vi "Pr650_K2400_Measure09.vi"(5 "error in":errorcluster, 6 "Volt":string, 7 "Device Name":string="OLED", 8 "Path":path=path "C:/temp", 9 "Keithly2400 Address":string, 10 "Port":i32(ring) items=["COM1", "COM2"]) -> (0 "error out(measure and off)":errorcluster, 1 "1931 CIE x":string, 2 "L: Cd/m^2":string, 3 "Keithley Data":string, 4 "1931 CIE y":string)   [LabVIEW 2009]
panel:
  in  "分支常量\n（见即时帮助）":bool
  out "string read":string
  out "error out(setup and on)":errorcluster
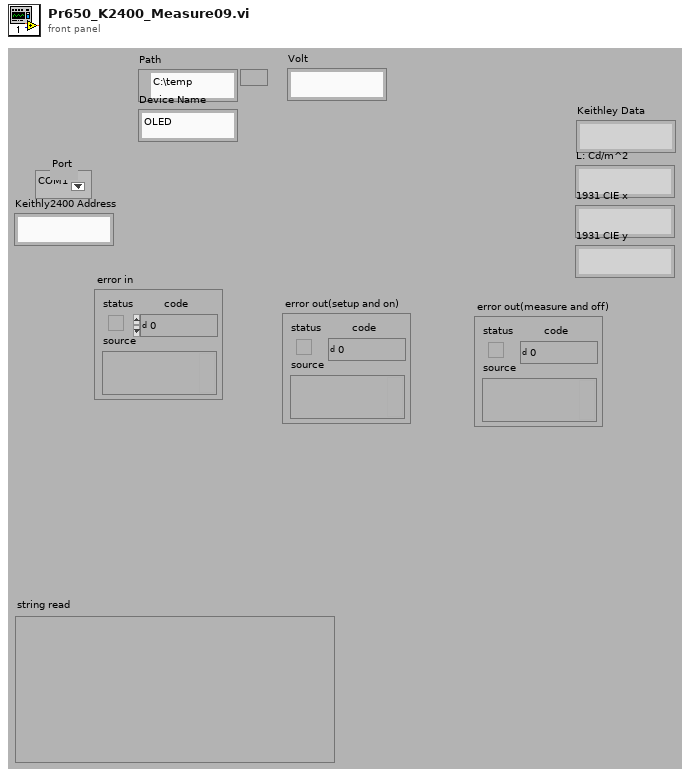
[diagram p1: front panel]
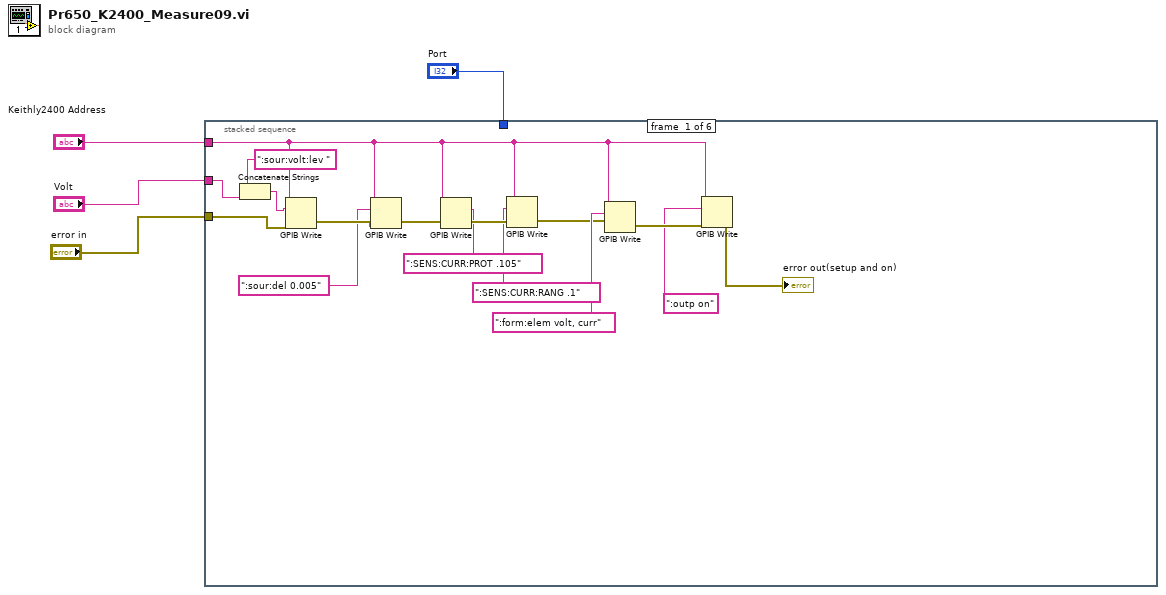
[diagram p0: block diagram]
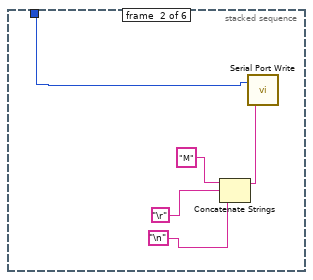
[diagram p2: hidden frame]
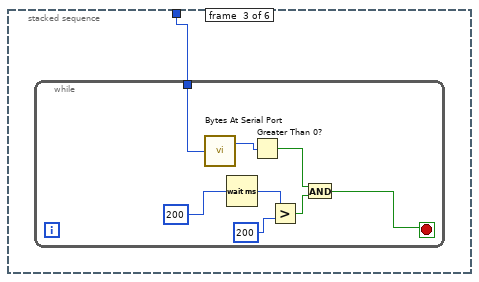
[diagram p3: hidden frame]
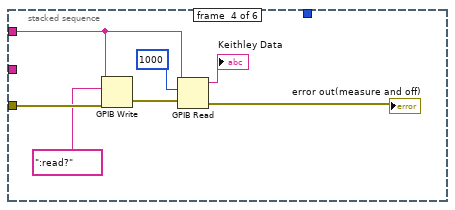
[diagram p4: hidden frame]
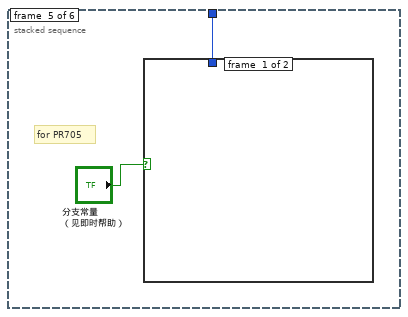
[diagram p5: hidden frame]
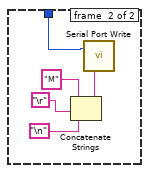
[diagram p6: hidden frame]
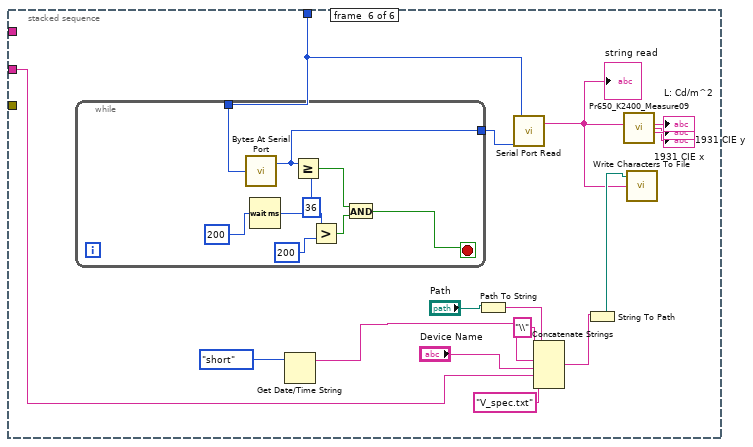
[diagram p7: hidden frame]
diagram:
  n1 = stacked-sequence {
    tunnel: "Port" -> [_ w22 w26 _ w43 w51]
    tunnel: "error in" -> [w20 _ _ w41 _ _]
    tunnel: "Keithly2400 Address" -> [w10 _ _ w36 _ _]
    tunnel: "Volt" -> [w14 _ _ _ _ w54]
    frame #0 {
      n2 = Concatenate Strings(":sour:volt:lev ", w14) -> (w12:string)
      n3 = GPIB Write(0:w10, 1:w12, 3:w20) -> (6:w19:errorcluster)  [unwired: 2 in, 1 out]
      n4 = GPIB Write(0:w10, 1:":sour:del 0.005" ("data"), 3:w19) -> (6:w9:errorcluster)  [unwired: 2 in, 1 out]
      n5 = GPIB Write(0:w10, 1:":SENS:CURR:PROT .105", 3:w9) -> (6:w8:errorcluster)  [unwired: 2 in, 1 out]
      n6 = GPIB Write(0:w10, 1:":SENS:CURR:RANG .1", 3:w8) -> (6:w7:errorcluster)  [unwired: 2 in, 1 out]
      n7 = GPIB Write(0:w10, 1:":form:elem volt, curr" ("data"), 3:w7) -> (6:w16:errorcluster)  [unwired: 2 in, 1 out]
      n8 = GPIB Write(0:w10, 1:":outp on" ("data"), 3:w16) -> (6:→"error out(setup and on)":errorcluster)  [unwired: 2 in, 1 out]
    }
    frame #1 {
      n9 = Concatenate Strings("M" ("string"), "\r", "\n") -> (w25:string)
      n10 = call <vilib>:"Serial Port Write.vi"("string to write"=w25, "port number"=w22) -> ()  [unwired: 1 out]
    }
    frame #2 {
      n11 = while {
        tunnel: w26 -> [w33]
        stop <- w28 stop-if-true
        n12 = call <vilib>:"Bytes At Serial Port.vi"("port number"=w33) -> ("byte count"=w27:u32)  [unwired: 1 out]
        n13 = Wait (ms)(milliseconds to wait=u32 200) -> (millisecond timer value=w31:u32)
        n14 = Greater Than 0?(x=w27) -> (x > 0?=w29:bool)
        n15 = Greater?(x=w31, y=u32 200) -> (0:w32:bool)
        n16 = And(x=w29, y=w32) -> (x .and. y?=w28:bool)
      }
    }
    frame #3 {
      n17 = GPIB Write(0:w36, 1:":read?" ("data"), 3:w41) -> (6:w39:errorcluster)  [unwired: 2 in, 1 out]
      n18 = GPIB Read(0:w36, 1:1000 ("byte count"), 3:w39) -> (5:→"Keithley Data":string, 7:→"error out(measure and off)":errorcluster)  [unwired: 2 in, 1 out]
    }
    frame #4 {
      # "for PR705"
      n19 = case shown="真" "分支常量\n（见即时帮助）" {
        tunnel: w43 -> [_ w45]
        frame #0 {
        }
        frame #1 {
          n20 = Concatenate Strings("M" ("string"), "\r", "\n") -> (w46:string)
          n21 = call <vilib>:"Serial Port Write.vi"("string to write"=w46, "port number"=w45) -> ()  [unwired: 1 out]
        }
      }
    }
    frame #5 {
      n22 = while {
        tunnel: [w65] -> w52
        tunnel: w51 -> [w72]
        stop <- w67 stop-if-true
        n23 = call <vilib>:"Bytes At Serial Port.vi"("port number"=w72) -> ("byte count"=w65:u32)  [unwired: 1 out]
        n24 = Wait (ms)(milliseconds to wait=u32 200) -> (millisecond timer value=w70:u32)
        n25 = Greater Or Equal?(x=w65, y=u32 36) -> (x >= y?=w68:bool)
        n26 = Greater?(x=w70, y=u32 200) -> (0:w71:bool)
        n27 = And(x=w68, y=w71) -> (x .and. y?=w67:bool)
      }
      n28 = Get Date/Time String(date format (0)=enum16{"short", "long", "abbreviated"}."short") -> (date string=w49:string)  [unwired: 2 in, 1 out]
      n29 = Path To String(path="Path") -> (string=w63:string)
      n30 = call <vilib>:"Serial Port Read.vi"("requested byte count"=w52, "port number"=w51) -> ("string read"=w50:string)  [unwired: 1 out]
      "string read" <- w50
      n31 = Concatenate Strings(w63, "\\" ("Substring"), w49, "Device Name", w54, "V_spec.txt") -> (w64:string)
      n32 = String To Path(string=w64) -> (path=w61:path)
      n33 = call "Pr650_K2400_Measure09.vi"("Keithly2400 Address"=w50) -> ("1931 CIE x"=→"1931 CIE x":string, "L: Cd/m^2"=→"L: Cd/m^2":string, "1931 CIE y"=→"1931 CIE y":string)  [unwired: 5 in, 2 out]
      n34 = call <vilib>:"Write Characters To File.vi"("character string"=w50, "file path (dialog if empty)"=w61) -> ()  [unwired: 3 in, 1 out]
    }
  }
